vi "XDataNode9_0To8_6.vi"(10 "Version-State Cluster In":T1, 11 "XRef":refnum<vi>) -> (0 "Custom Label":string, 1 "Custom Warning To Issue":string, 2 "Version-State Cluster Out":T1, 3 "Action":T2)   [LabVIEW 2020]
uses:
  <vilib>/XSFPSupport/SFPChangeStateAction.ctl
  <vilib>/XNodeSupport/XNodeVersion.ctl
  <vilib>/XNodeSupport/XNodeUShort.ctl
  <vilib>/Platform/TimedLoop/XDataNode/XDataNode.ctl
  <vilib>/Platform/TimedLoop/XDataNode/timing_clust.ctl
  <vilib>/Platform/TimedLoop/XDataNode/nitl_modes.ctl
  <vilib>/Platform/TimedLoop/XDataNode/wakeup.ctl
  <vilib>/Platform/TimedLoop/XDataNode/TermInfo.ctl
  <vilib>/Platform/TimedLoop/XDataNode/nitl_TargetSpecificData.ctl
  <vilib>/Platform/TimedLoop/XDataNode/DN_Type.ctl
  <vilib>/XSFPSupport/NI_XSFPSupport.lvlib
  <vilib>/XNodeSupport/NI_XNodeSupport.lvlib
  <vilib>/Platform/TimedLoop/XDataNode/XDataNode.xnode
  <vilib>/Platform/TimedLoop/XDataNode/XDNodeRunTimeDep.lvlib
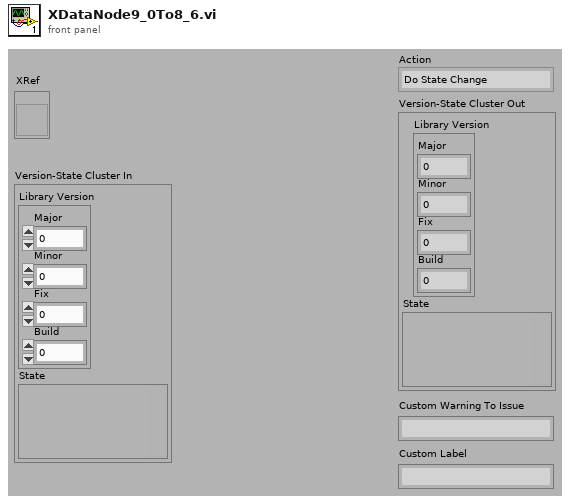
[diagram p1: front panel]
types:
  T1 = cluster{"Library Version":cluster{"Major":u16, "Minor":u16, "Fix":u16, "Build":u16}, "State":variant}
  T2 = typedef "NI_XSFPSupport.lvlib/SFPChangeStateAction.ctl" = enum32{"Do State Change", "Replace With Label", "Fail SFP"}
  T3 = typedef "XDataNode.xnode/XDataNode.ctl" = cluster{"Timing":T4, "Size":T7[], "Hidden":T7[], "Invisible":bool[], "Input?":bool, "timing src wired?":bool, "Target Specific Data":T8[], "G Only Data":variant, "DataNode_Type":T9}
  T4 = typedef "XDNodeRunTimeDep.lvlib/timing_clust.ctl" = cluster{"Expected End [f-1]":u64, "Actual End [f-1]":u64, "Finished Late? [f-1]":bool, "Expected End [i-1]":u64, "Actual End [i-1]":u64, "Finished Late? [i-1]":bool, "Expected Start [i]":u64, "Actual Start [i]":u64, "Expected Start [f]":u64, "Actual Start [f]":u64, "Source Name":string, "Structure Name":string, "Period":i64, "Deadline":i64, "Offset":i64, "Start":i64, "Priority":i32, "Timeout":i32, "Mode":T5, "Wakeup Reason":T6, "Error":errorcluster, "Source Type":string, "Secondary Source Type":string, "Global End Time":u64, "Global Start Time":u64, "Frame Duration":u64, "Iteration Duration":u64, "Assigned CPU":i32, "I/O Scan Engine Mode":u32}
  T5 = typedef "XDNodeRunTimeDep.lvlib/nitl_modes.ctl" = enum32{"No Change", "Process missed periods, maintain original phase", "Discard missed periods, maintain original phase", "Process missed periods, ignore original phase", "Discard missed periods, ignore original phase"}
  T6 = typedef "XDNodeRunTimeDep.lvlib/wakeup.ctl" = enum32{"Normal", "Aborted", "Asynchronous wakeup", "Timing source error", "Timed loop error", "Timeout"}
  T7 = typedef "XDataNode.xnode/TermInfo.ctl" = cluster{"ID":i32, "Wired?":bool, "Type":variant, "Name":string, "Input?":bool, "StaticID":i32}
  T8 = typedef "XDataNode.xnode/nitl_TargetSpecificData.ctl" = cluster{"Target Name":string, "Target Data":variant}
  T9 = typedef "XDataNode.xnode/DN_Type.ctl" = enum32{"TL_Lft_Ear", "TL_Rt_Ear", "TL_Lft_Dn", "TL_Rt_Dn", "TS_Lft_Ear", "TS_Rt_Ear", "TS_1stFrame_Lft_Dn", "TS_Lft_Dn", "TS_LastFrame_Rt_Dn", "TS_Rt_Dn", "TL_TS_Lft_Ear", "TL_TS_Rt_Ear", "TL_TS_Lft_Dn", "TL_TS_Rt_Dn", "TL_TS_1stFrame_Lft_Dn", "TL_TS_LastFrame_Rt_Dn"}
  T10 = typedef "NI_XNodeSupport.lvlib/XNodeVersion.ctl" = cluster{"Major":T11, "Minor":T11, "Fix":T11, "Build":T11}
  T11 = typedef "NI_XNodeSupport.lvlib/XNodeUShort.ctl" = u16
  T12 = cluster{"Major":u16, "Minor":u16, "Fix":u16, "Build":u16}
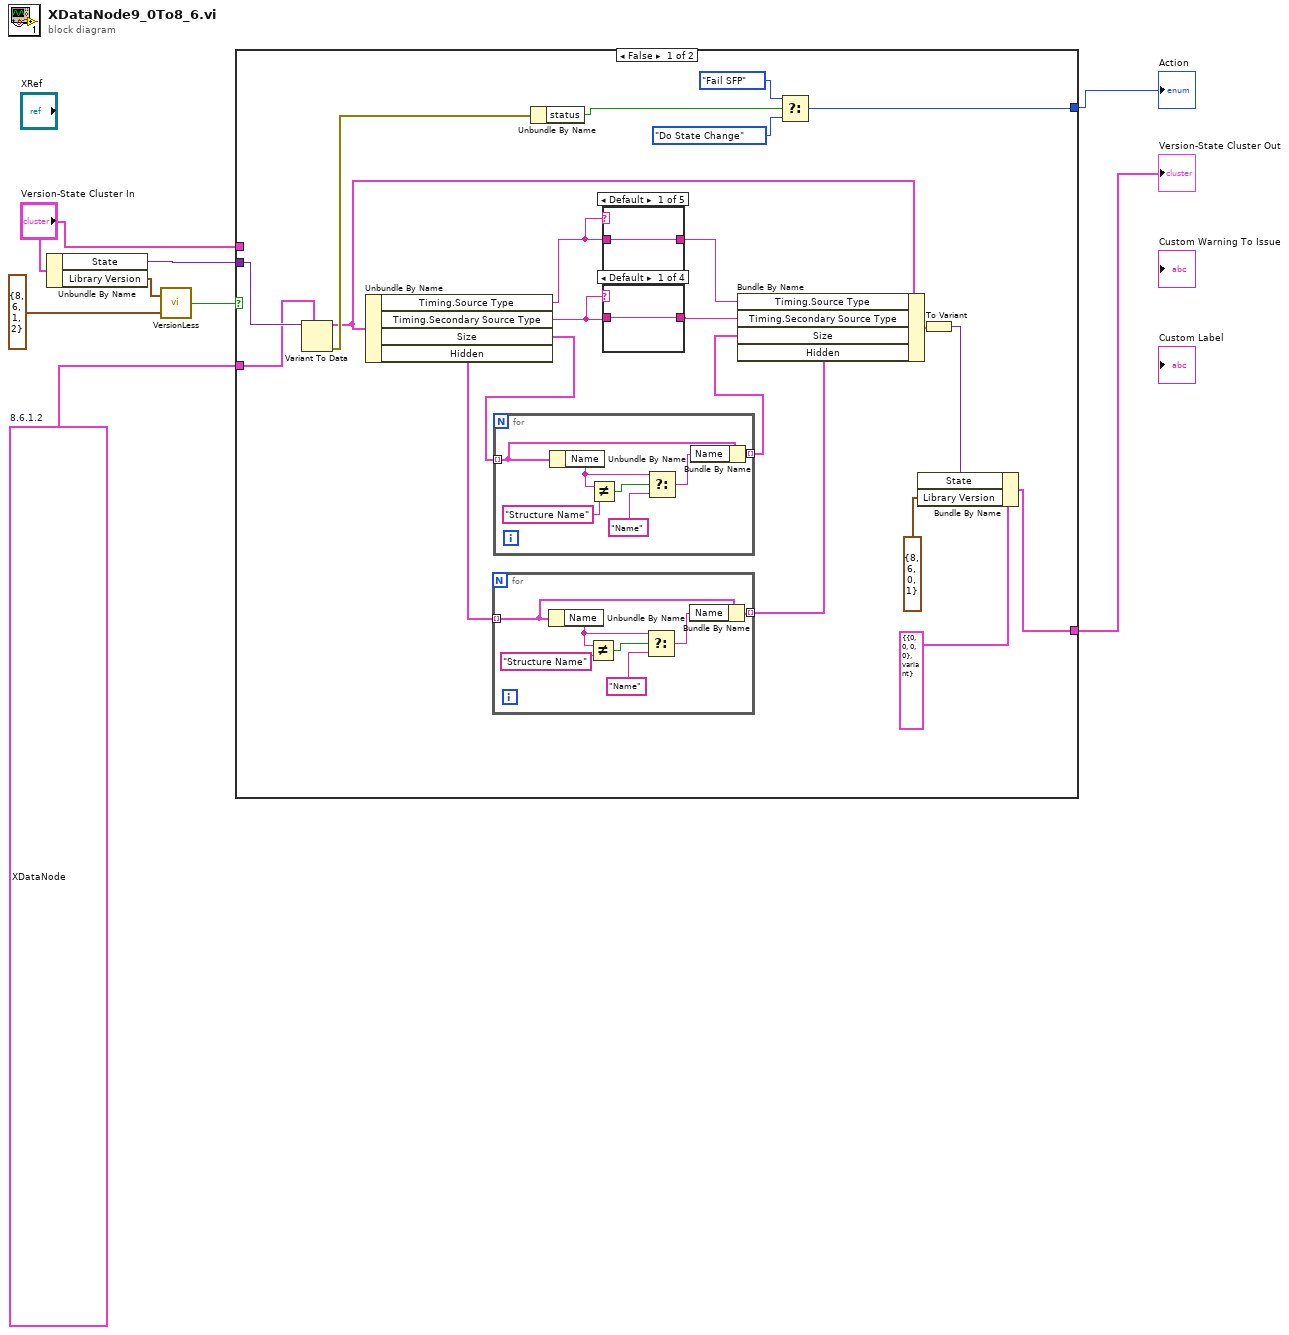
[diagram p0: block diagram]
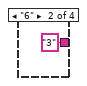
[diagram p2: hidden frame]
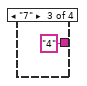
[diagram p3: hidden frame]
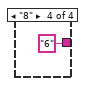
[diagram p4: hidden frame]
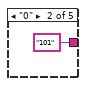
[diagram p5: hidden frame]
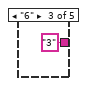
[diagram p6: hidden frame]
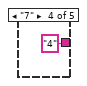
[diagram p7: hidden frame]
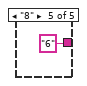
[diagram p8: hidden frame]
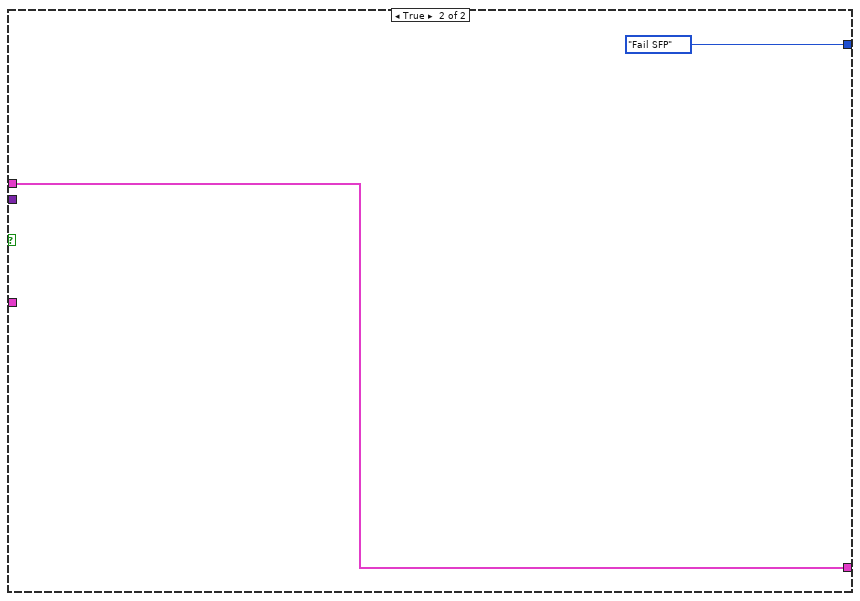
[diagram p9: hidden frame]
diagram:
  w3 = T3 {"Timing"={"Expected End [f-1]"=0, "Actual End [f-1]"=0, "Finished Late? [f-1]"=FALSE, "Expected End [i-1]"=0, "Actual End [i-1]"=0, "Finished Late? [i-1]"=FALSE, "Expected Start [i]"=0, "Actual Start [i]"=0, "Expected Start [f]"=0, "Actual Start [f]"=0, "Source Name"="", "Structure Name"="", "Period"=0, "Deadline"=0, "Offset"=0, "Start"=0, "Priority"=0, "Timeout"=0, "Mode"=enum."No Change", "Wakeup Reason"=enum."Normal", "Error"={"status"=FALSE, "code"=0, "source"=""}, "Source Type"="", "Secondary Source Type"="", "Global End Time"=0, "Global Start Time"=0, "Frame Duration"=0, "Iteration Duration"=0, "Assigned CPU"=0, "I/O Scan Engine Mode"=0}, "Size"=[], "Hidden"=[], "Invisible"=[], "Input?"=FALSE, "timing src wired?"=FALSE, "Target Specific Data"=[], "G Only Data"=variant, "DataNode_Type"=enum."TL_Lft_Ear"}  # 8.6.1.2
  n1 = Unbundle By Name("Version-State Cluster In") -> ("State"=w4:variant, "Library Version"=w5:T12)
  n2 = call <vilib>:"VersionLess.vi"("y"=T10 {"Major"=8, "Minor"=6, "Fix"=1, "Build"=2}, "x"=w5) -> ("x < y?"=w7:bool)
  n3 = case shown="False" w7 {
    tunnel: [w23 SFPChangeStateAction."Fail SFP" ("Action")] -> w6
    tunnel: w4 -> [w29 _]
    tunnel: w3 -> [w28 _]
    tunnel: [w18 w53] -> w2
    tunnel: "Version-State Cluster In" -> [_ w53]
    frame False {
      n4 = Variant To Data(type=w28, Variant=w29) -> (data=w17:T3, error out=w27:errorcluster)  [unwired: 1 in]
      n5 = Unbundle By Name(w17) -> ("Timing.Source Type"=w11:string, "Timing.Secondary Source Type"=w9:string, "Size"=w15:T7[], "Hidden"=w13:T7[])
      n6 = for {
        tunnel: w13 -> [w36] mode=indexing
        tunnel: [w35] -> w12 mode=indexing
        n7 = Unbundle By Name(w36) -> ("Name"=w38:string)
        n8 = Not Equal?(x=w38, y="Structure Name") -> (x != y?=w39:bool)
        n9 = Select(t=w38, s=w39, f="Name") -> (s? t:f=w34:string)
        n10 = Bundle By Name(cluster=w36, "Name"=w34) -> (w35:T7)
      }
      n11 = for {
        tunnel: w15 -> [w43] mode=indexing
        tunnel: [w42] -> w14 mode=indexing
        n12 = Unbundle By Name(w43) -> ("Name"=w45:string)
        n13 = Not Equal?(x=w45, y="Structure Name") -> (x != y?=w46:bool)
        n14 = Select(t=w45, s=w46, f="Name") -> (s? t:f=w41:string)
        n15 = Bundle By Name(cluster=w43, "Name"=w41) -> (w42:T7)
      }
      n16 = Unbundle By Name(w27) -> ("status"=w26:bool)
      n17 = case shown="Default" w11 {
        tunnel: [w48 "101" ("Source Type") "3" "4" "6"] -> w16
        tunnel: w11 -> [w48 _ _ _ _]
        frame Default {
        }
        frame "0" {
        }
        frame "6" {
        }
        frame "7" {
        }
        frame "8" {
        }
      }
      n18 = case shown="Default" w9 {
        tunnel: [w30 "3" "4" "6"] -> w10
        tunnel: w9 -> [w30 _ _ _]
        frame Default {
        }
        frame "6" {
        }
        frame "7" {
        }
        frame "8" {
        }
      }
      n19 = Bundle By Name(cluster=w17, "Timing.Source Type"=w16, "Timing.Secondary Source Type"=w10, "Size"=w14, "Hidden"=w12) -> (w22:T3)
      n20 = Select(t=SFPChangeStateAction."Fail SFP" ("Action"), s=w26, f=SFPChangeStateAction."Do State Change" ("Action")) -> (s? t:f=w23:T2)
      n21 = To Variant(anything=w22) -> (Variant=w19:variant)
      n22 = Bundle By Name(cluster=T1 {"Library Version"={"Major"=0, "Minor"=0, "Fix"=0, "Build"=0}, "State"=variant} ("Version-State Cluster Out"), "State"=w19, "Library Version"=T10 {"Major"=8, "Minor"=6, "Fix"=0, "Build"=1} ("y")) -> (w18:T1)
    }
    frame True {
    }
  }
  "Action" <- w6
  "Version-State Cluster Out" <- w2
